vi "FGV_Dialog_Boolean.vi"(0 "Boolean In":bool, 7 "Action":enum16{"Write", "Read"}(ring), 11 "Error In":errorcluster) -> (4 "Boolean Out":bool, 15 "Error Out":errorcluster)   [LabVIEW 2016]
doc: "This VI gets or sets the GEA2 reference."
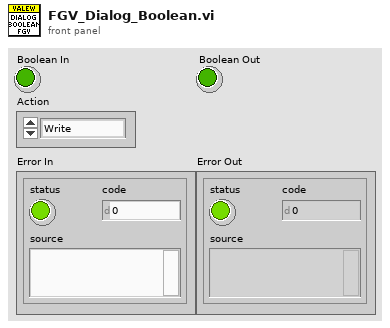
[diagram p1: front panel]
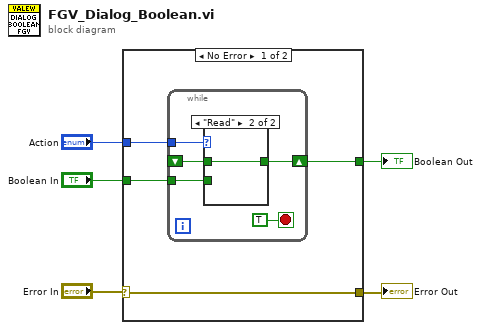
[diagram p0: block diagram]
diagram:
  n1 = case shown="No Error" "Error In" {
    selector: "Error In" -> [w6 w17]
    tunnel: "Action" -> [w9 _]
    tunnel: "Boolean In" -> [w8 _]
    tunnel: [w7 _] -> w3
    tunnel: [w6 w17] -> w1
    frame No Error {
      n2 = while {
        tunnel: w9 -> [w13]
        tunnel: w8 -> [w12]
        shift-right: [w11] -> w7
        shift-left: _ -> [w10]
        stop <- TRUE stop-if-true
        n3 = case shown="\"Read\"" w13 {
          tunnel: w12 -> [w15 _]
          tunnel: [w15 w16] -> w11
          tunnel: w10 -> [_ w16]
          frame "Write" {
          }
          frame "Read" {
          }
        }
      }
    }
    frame Error {
    }
  }
  "Boolean Out" <- w3
  "Error Out" <- w1
